vi "File list dialog.vi"(10 "Filters":string[](array[string])=["All files (*.*)|*.*"], 11 "File list in":path[](array[path])) -> (2 "Canceled?":bool, 3 "File list out":path[](array[path]))   [LabVIEW 2011, in "COSYLib.lvlib"]
doc: "Lets the user select a set of files.\nTo let the user select files of a specific type, use the <B>Filters</B> terminal. This is an array of strings of the format \"My Files (*.my)|*.my\"."
uses:
  COSYLib.lvlib
  <vilib>/Utility/miscctls.llb/LVPointTypeDef.ctl
panel:
  in  "Browse button":bool
  in  "Files of type:":string(combo)
  in  "Remove file":bool
  in  "Remove all":bool
  in  "Add all":bool
  in  "Add file":bool
  in  "Files":i32[](listbox)
  in  "Path":path
  in  "Selected files":i32[](listbox)
  out "Resized?":bool
  in  "Cancel":bool
  in  "OK":bool
  # "File Browser"
  # "Selected Files"
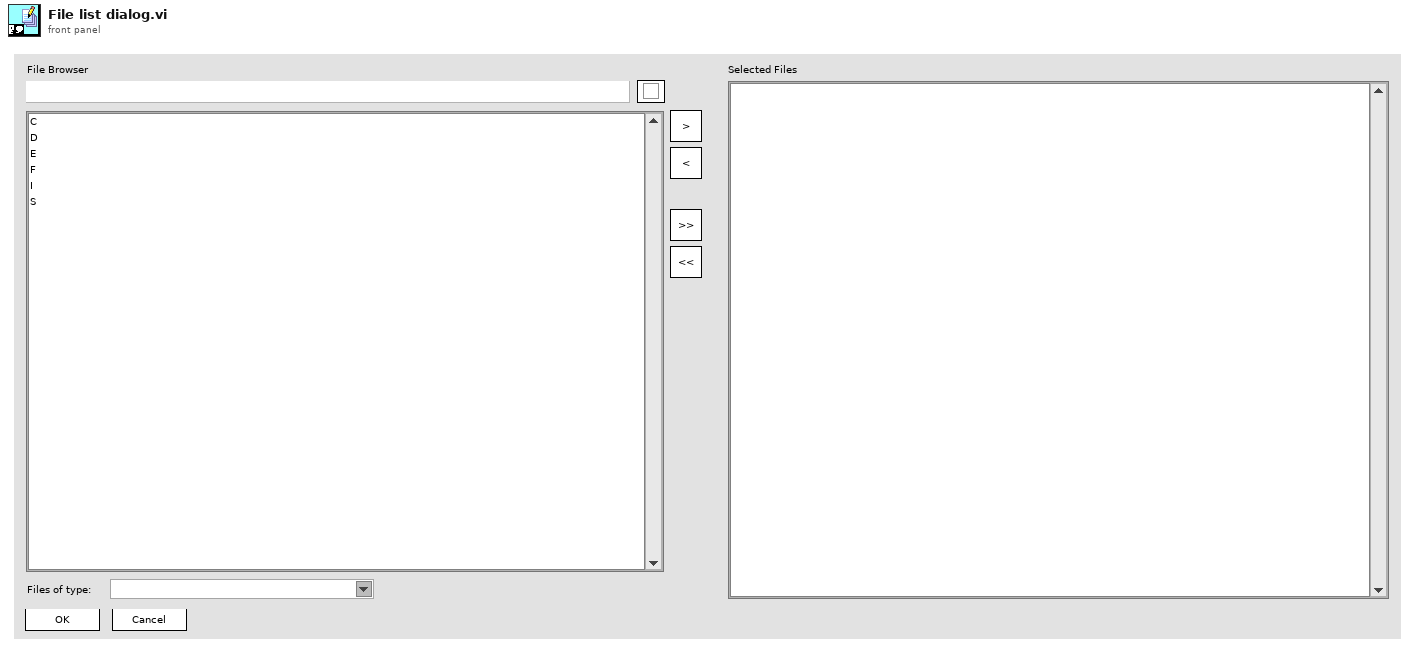
[diagram p1: front panel]
types:
  T1 = typedef "eventvkey.ctl" = enum16{"ASCII", "Enter", "Return", "Shift", "Ctrl", "Alt", "Cmd", "Opt", "Caps", "NumLock", "Clear", "Break", "Up", "Down", "Left", "Right", "Insert", "Delete", "Home", "End", "PageUp", "PageDown", "Escape", "Help", "Pause", "ScrollLock", "F1", "F2", "F3", "F4", "F5", "F6", "F7", "F8", "F9", "F10", "F11", "F12", "F13", "F14", "F15", "F16", "F17", "F18", "F19", "F20", "F21", "F22", "F23", "F24", "Play", "VolumeUp", "VolumeDown", "Mute", "Two Byte Char"}
  T2 = typedef "LVPointTypeDef.ctl" = cluster{"Horizontal":i16, "Vertical":i16}
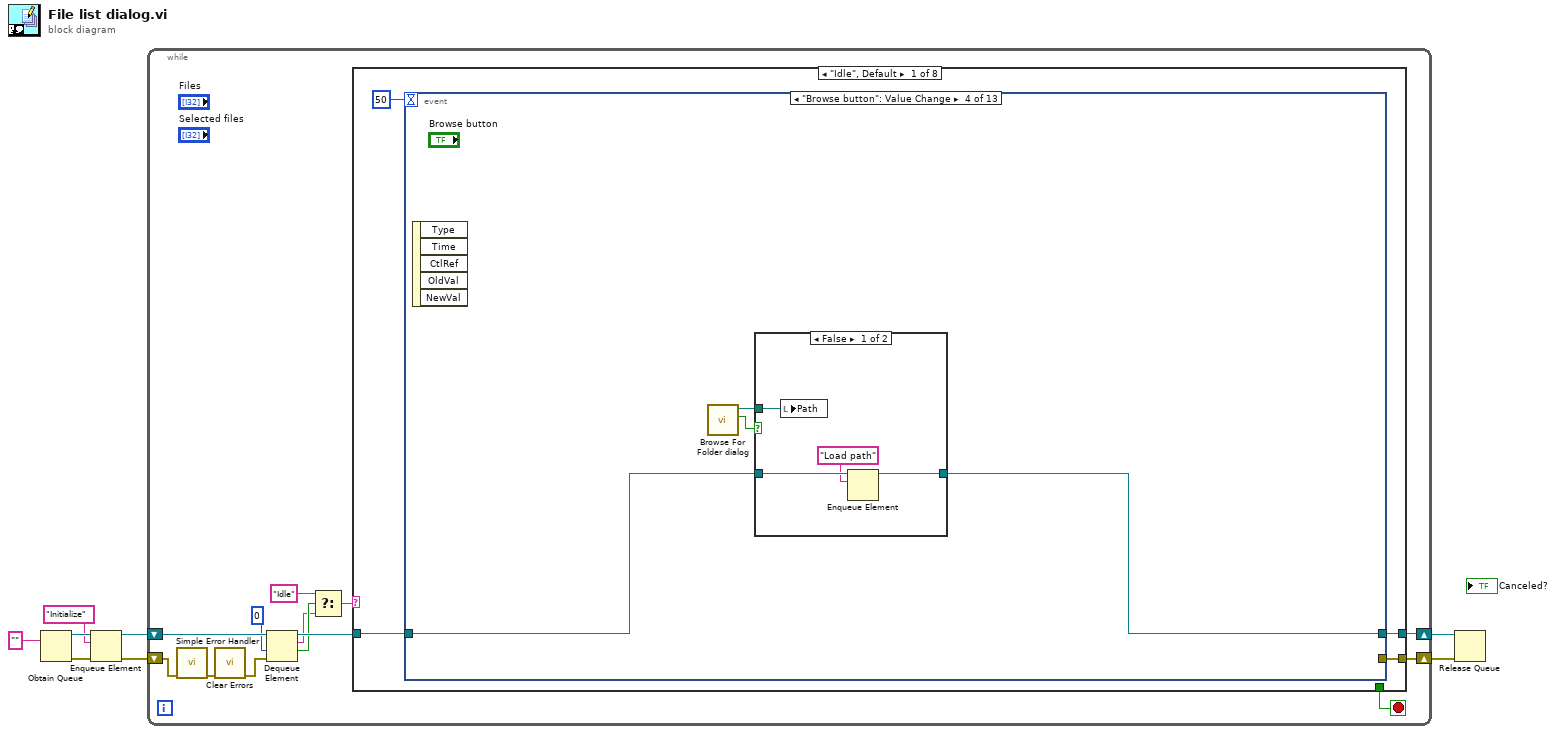
[diagram p0: block diagram]
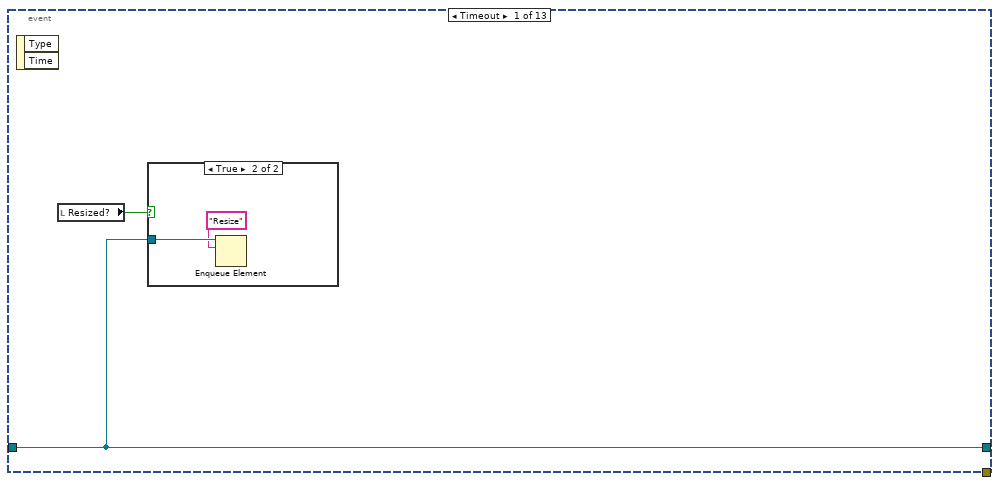
[diagram p2: hidden frame]
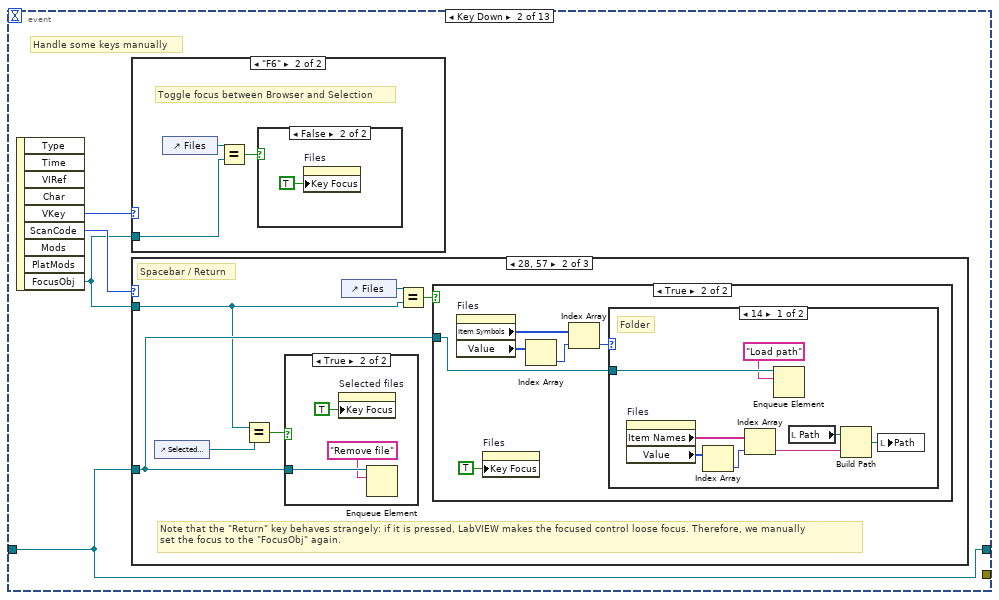
[diagram p4: hidden frame]
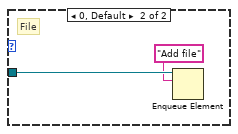
[diagram p8: hidden frame]
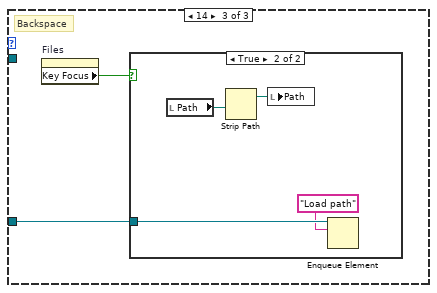
[diagram p9: hidden frame]
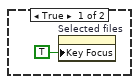
[diagram p12: hidden frame]
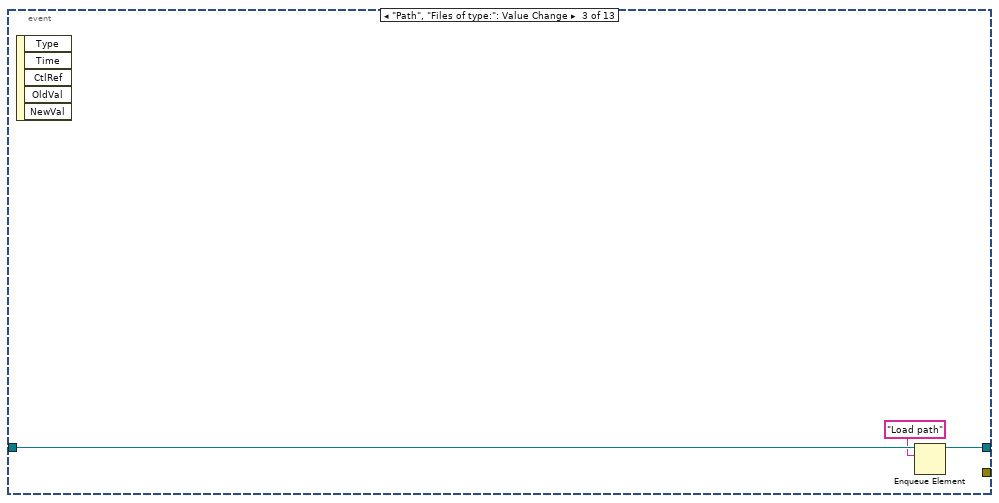
[diagram p13: hidden frame]
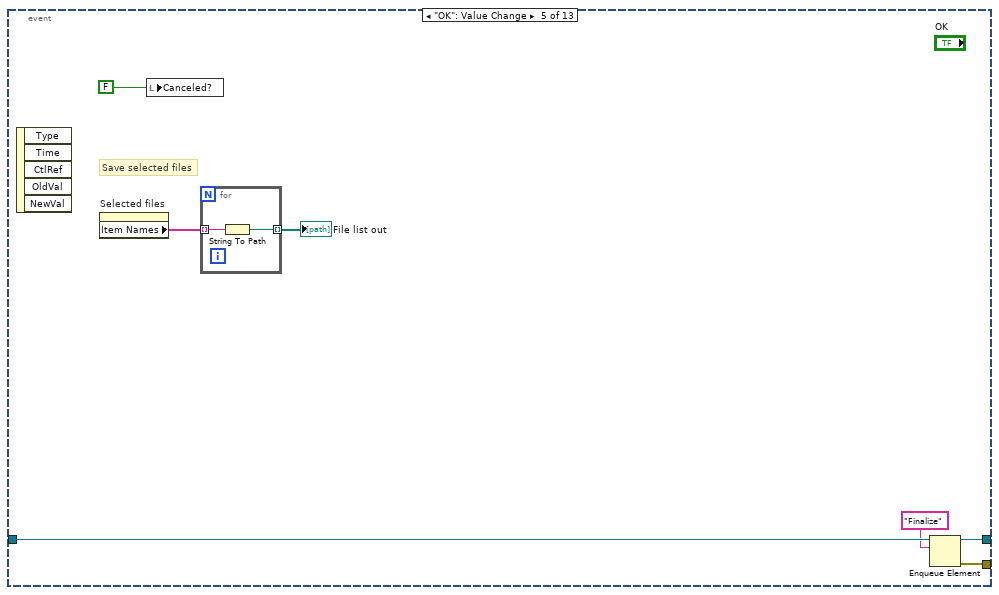
[diagram p15: hidden frame]
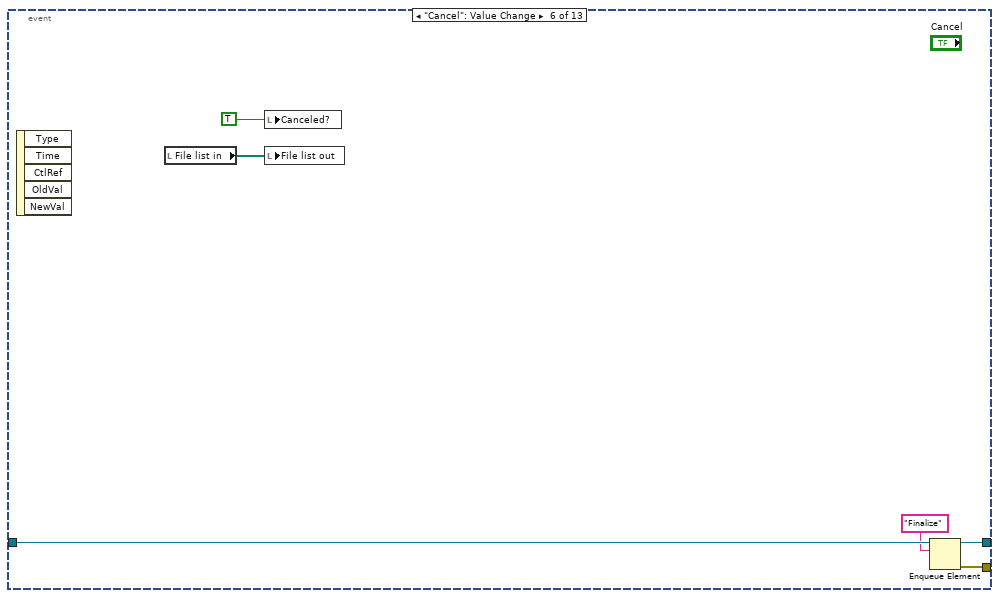
[diagram p16: hidden frame]
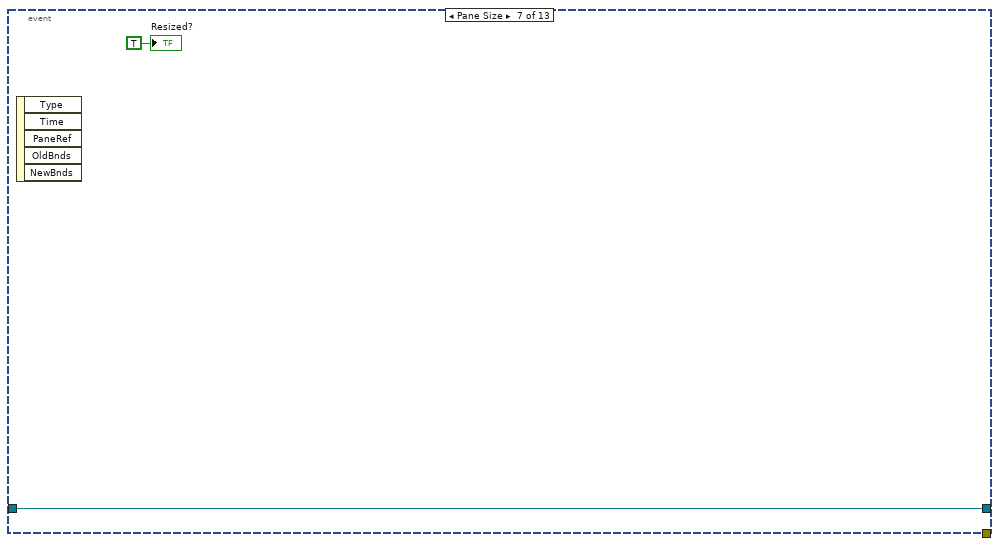
[diagram p17: hidden frame]
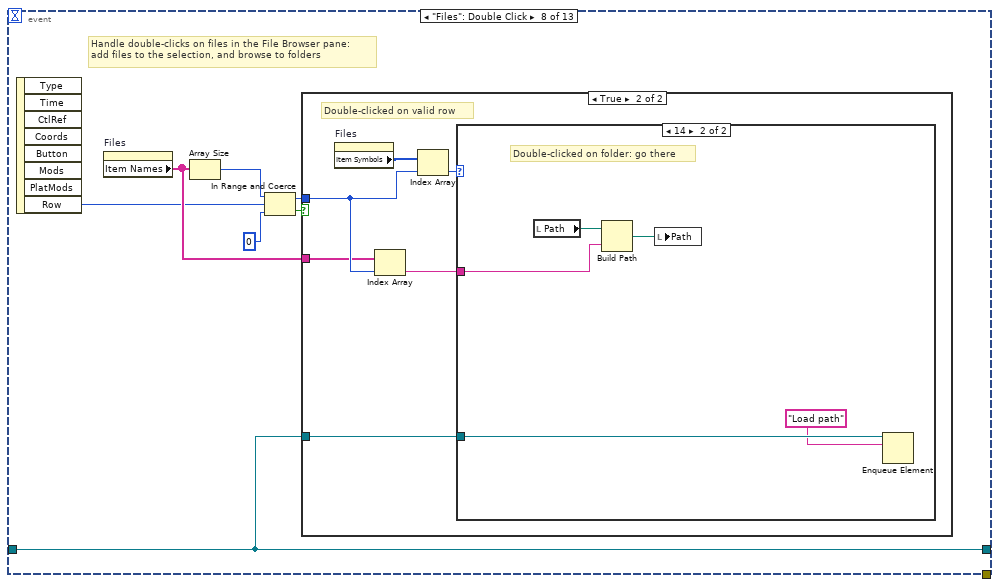
[diagram p18: hidden frame]
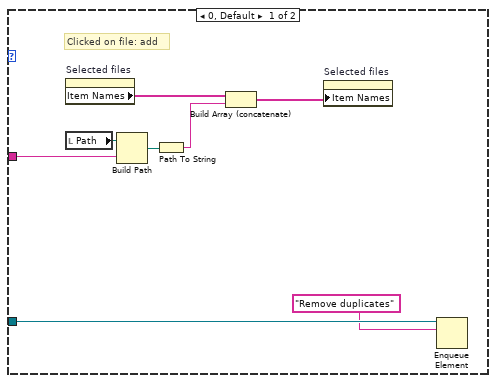
[diagram p20: hidden frame]
diagram:
  n1 = Obtain Queue(element data type="") -> (queue out=w7:refnum<queue>, error out=w6:errorcluster)  [unwired: 4 in, 1 out]
  n2 = Enqueue Element(queue=w7, element="Initialize", error in (no error)=w6) -> (queue out=w4:refnum<queue>, error out=w3:errorcluster)  [unwired: 1 in, 1 out]
  n3 = while {
    shift-right: [w10] -> w2
    shift-left: w3 -> [w20]
    shift-right: [w9] -> w1
    shift-left: w4 -> [w19]
    stop <- w21 stop-if-true
    n4 = call <vilib>:"Simple Error Handler.vi"("error in (no error)"=w20) -> ("error out"=w12:errorcluster)  [unwired: 4 in, 4 out]
    n5 = call <vilib>:"Clear Errors.vi"("error in (no error)"=w12) -> ("error out"=w11:errorcluster)  [unwired: 6 in]
    n6 = Dequeue Element(queue=w19, timeout in ms (-1)=0, error in (no error)=w11) -> (queue out=w17:refnum<queue>, element=w14:string, timed out?=w15:bool)  [unwired: 1 out]
    n7 = Select(t="Idle", s=w15, f=w14) -> (s? t:f=w18:string)
    n8 = case shown="\"Idle\", Default" w18 {
      tunnel: [_ _ TRUE _ _ _ _ _] -> w21
      tunnel: w17 -> [w25 w187 w199 w204 w231 w258 w284 w290]
      tunnel: [w24 _ _ _ _ _ _ _] -> w10
      tunnel: [w22 w177 w199 w204 w231 w249 w284 w290] -> w9
      frame "Idle", Default {
        n9 = event shown="[3] \"Browse button\": Value Change" {
          selector: _ -> [_ _ _ _ _ _ _ _ _ _ _ _ _]
          dyn-events: _ -> [_ _ _ _ _ _ _ _ _ _ _ _ _]
          timeout: 50 -> [_ _ _ _ _ _ _ _ _ _ _ _ _]
          tunnel: w25 -> [w26 w31 w72 w76 w88 w93 w98 w99 w131 w136 w146 w166 w169]
          tunnel: [_ _ _ _ w86 w95 _ _ _ _ _ _ _] -> w24
          tunnel: [w26 w31 w71 w75 w84 w94 w98 w99 w131 w136 w138 w165 w168] -> w22
          event Timeout {
            n10 = event-data() -> ()  [unwired: 1 in, 2 out]
            n11 = local read "Resized?"() -> (w27:bool)
            n12 = case shown="True" w27 {
              tunnel: w26 -> [_ w29]
              frame False {
              }
              frame True {
                n13 = Enqueue Element(queue=w29, element="Resize") -> ()  [unwired: 2 in, 3 out]
              }
            }
          }
          event Key Down {
            # "Handle some keys manually"
            n14 = event-data() -> ("VKey"=w33:T1, "ScanCode"=w32:i16, "FocusObj"=w30:refnum<vi>)  [unwired: 1 in, 6 out]
            n15 = case shown="\"F6\"" w33 {
              tunnel: w30 -> [_ w65]
              frame Default {
              }
              frame "F6" {
                # "Toggle focus between Browser and Selection"
                n16 = control-ref of="Files"() -> (w67:refnum<vi>)
                n17 = Equal?(x=w67, y=w65) -> (x = y?=w66:bool)
                n18 = case shown="False" w66 {
                  frame True {
                    n19 = property on="Selected files" class="LstBox (strict)"("Key Focus"=TRUE) -> ()  [unwired: 2 in, 2 out]
                  }
                  frame False {
                    n20 = property on="Files" class="LstBox (strict)"("Key Focus"=TRUE) -> ()  [unwired: 2 in, 2 out]
                  }
                }
              }
            }
            n21 = case shown="28, 57" w32 {
              tunnel: w31 -> [_ w39 w59]
              tunnel: w30 -> [_ w34 _]
              frame Default {
              }
              frame 28, 57 {
                # "Note that the \"Return\" key behaves strangely: if it is pressed, LabVIEW makes the focused control loose focus. Therefore, we manually\nset the focus to the \"FocusObj\" again."
                # "Spacebar / Return"
                n22 = control-ref of="Selected files"() -> (w35:refnum<vi>)
                n23 = Equal?(x=w34, y=w35) -> (x = y?=w36:bool)
                n24 = case shown="True" w36 {
                  tunnel: w39 -> [_ w42]
                  frame False {
                  }
                  frame True {
                    n25 = property on="Selected files" class="LstBox (strict)"("Key Focus"=TRUE) -> ()  [unwired: 2 in, 2 out]
                    n26 = Enqueue Element(queue=w42, element="Remove file") -> ()  [unwired: 2 in, 3 out]
                  }
                }
                n27 = control-ref of="Files"() -> (w37:refnum<vi>)
                n28 = Equal?(x=w37, y=w34) -> (x = y?=w38:bool)
                n29 = case shown="True" w38 {
                  tunnel: w39 -> [_ w46]
                  frame False {
                  }
                  frame True {
                    n30 = property on="Files" class="LstBox (strict)"() -> ("Item Symbols"=w48:i32[], "Value"=w45:i32[])  [unwired: 2 in, 2 out]
                    n31 = property on="Files" class="LstBox (strict)"("Key Focus"=TRUE) -> ()  [unwired: 2 in, 2 out]
                    n32 = Index Array(array=w45) -> (element=w44:i32)  [unwired: 1 in]
                    n33 = Index Array(array=w48, index=w44) -> (element=w47:i32)
                    n34 = case shown="14" w47 {
                      tunnel: w46 -> [w56 w58]
                      frame 14 {
                        # "Folder"
                        n35 = property on="Files" class="LstBox (strict)"() -> ("Item Names"=w52:string[], "Value"=w50:i32[])  [unwired: 2 in, 2 out]
                        n36 = Index Array(array=w50) -> (element=w49:i32)  [unwired: 1 in]
                        n37 = Index Array(array=w52, index=w49) -> (element=w51:string)
                        n38 = Enqueue Element(queue=w56, element="Load path") -> ()  [unwired: 2 in, 3 out]
                        n39 = local read "Path"() -> (w55:path)
                        n40 = Build Path(base path=w55, name or relative path=w51) -> (appended path=w54:path)
                        n41 = local write "Path"(w54) -> ()
                      }
                      frame 0, Default {
                        # "File"
                        n42 = Enqueue Element(queue=w58, element="Add file") -> ()  [unwired: 2 in, 3 out]
                      }
                    }
                  }
                }
              }
              frame 14 {
                # "Backspace"
                n43 = property on="Files" class="LstBox (strict)"() -> ("Key Focus"=w60:bool)  [unwired: 2 in, 2 out]
                n44 = case shown="True" w60 {
                  tunnel: w59 -> [_ w62]
                  frame False {
                  }
                  frame True {
                    n45 = local read "Path"() -> (w64:path)
                    n46 = Strip Path(path=w64) -> (stripped path=w63:path)  [unwired: 1 out]
                    n47 = local write "Path"(w63) -> ()
                    n48 = Enqueue Element(queue=w62, element="Load path") -> ()  [unwired: 2 in, 3 out]
                  }
                }
              }
            }
          }
          event "Path", "Files of type:": Value Change {
            n49 = event-data() -> ()  [unwired: 1 in, 5 out]
            n50 = Enqueue Element(queue=w72, element="Load path") -> (queue out=w71:refnum<queue>)  [unwired: 2 in, 2 out]
          }
          event "Browse button": Value Change {
            n51 = event-data() -> ()  [unwired: 1 in, 5 out]
            n52 = call "Browse For Folder dialog.vi"() -> ("Cancelled?"=w74:bool, "Selected path"=w73:path)  [unwired: 9 in, 1 out]
            n53 = case shown="False" w74 {
              tunnel: w76 -> [w80 w81]
              tunnel: [w79 w81] -> w75
              tunnel: w73 -> [w77 _]
              frame False {
                n54 = local write "Path"(w77) -> ()
                n55 = Enqueue Element(queue=w80, element="Load path") -> (queue out=w79:refnum<queue>)  [unwired: 2 in, 2 out]
              }
              frame True {
              }
            }
          }
          event "OK": Value Change {
            # "Save selected files"
            n56 = event-data() -> ()  [unwired: 1 in, 5 out]
            n57 = property on="Selected files" class="LstBox (strict)"() -> ("Item Names"=w83:string[])  [unwired: 2 in, 2 out]
            n58 = local write "Canceled?"(FALSE ("Canceled?")) -> ()
            n59 = for {
              tunnel: w83 -> [w90] mode=indexing
              tunnel: [w89] -> w82 mode=indexing
              n60 = String To Path(string=w90) -> (path=w89:path)
            }
            "File list out" <- w82
            n61 = Enqueue Element(queue=w88, element="Finalize") -> (queue out=w84:refnum<queue>, error out=w86:errorcluster)  [unwired: 2 in, 1 out]
          }
          event "Cancel": Value Change {
            n62 = event-data() -> ()  [unwired: 1 in, 5 out]
            n63 = local read "File list in"() -> (w91:path[])
            n64 = local write "Canceled?"(TRUE ("Canceled?")) -> ()
            n65 = local write "File list out"(w91) -> ()
            n66 = Enqueue Element(queue=w93, element="Finalize") -> (queue out=w94:refnum<queue>, error out=w95:errorcluster)  [unwired: 2 in, 1 out]
          }
          event Pane Size {
            n67 = event-data() -> ()  [unwired: 1 in, 5 out]
            "Resized?" <- TRUE ("Resized?")
          }
          event "Files": Double Click {
            # "Handle double-clicks on files in the File Browser pane:\nadd files to the selection, and browse to folders"
            n68 = event-data() -> ("Row"=w100:i32)  [unwired: 1 in, 7 out]
            n69 = property on="Files" class="LstBox (strict)"() -> ("Item Names"=w102:string[])  [unwired: 2 in, 2 out]
            n70 = Array Size(array=w102) -> (size(s)=w101:i32)
            n71 = In Range and Coerce(upper limit=w101, x=w100, lower limit=0 ("upper limit")) -> (coerced(x)=w104:i32, In Range?=w105:bool)
            n72 = case shown="True" w105 {
              tunnel: w104 -> [_ w109]
              tunnel: w102 -> [_ w108]
              tunnel: w99 -> [_ w106]
              frame False {
                # "Double-clicked on an invalid/empty row"
              }
              frame True {
                # "Double-clicked on valid row"
                n73 = property on="Files" class="LstBox (strict)"() -> ("Item Symbols"=w111:i32[])  [unwired: 2 in, 2 out]
                n74 = Index Array(array=w108, index=w109) -> (element=w107:string)
                n75 = Index Array(array=w111, index=w109) -> (element=w110:i32)
                n76 = case shown="14" w110 {
                  tunnel: w107 -> [w116 w123]
                  tunnel: w106 -> [w113 w121]
                  frame 0, Default {
                    # "Clicked on file: add"
                    n77 = property on="Selected files" class="LstBox (strict)"() -> ("Item Names"=w119:string[])  [unwired: 2 in, 2 out]
                    n78 = local read "Path"() -> (w117:path)
                    n79 = Build Path(base path=w117, name or relative path=w116) -> (appended path=w115:path)
                    n80 = Path To String(path=w115) -> (string=w114:string)
                    n81 = Build Array (concatenate)(w119, w114) -> (w118:string[])
                    n82 = property on="Selected files" class="LstBox (strict)"("Item Names"=w118) -> ()  [unwired: 2 in, 2 out]
                    n83 = Enqueue Element(queue=w113, element="Remove duplicates") -> ()  [unwired: 2 in, 3 out]
                  }
                  frame 14 {
                    # "Double-clicked on folder: go there"
                    n84 = local read "Path"() -> (w124:path)
                    n85 = Build Path(base path=w124, name or relative path=w123) -> (appended path=w122:path)
                    n86 = local write "Path"(w122) -> ()
                    n87 = Enqueue Element(queue=w121, element="Load path") -> ()  [unwired: 2 in, 3 out]
                  }
                }
              }
            }
          }
          event "Selected files": Double Click {
            # "Remove the file that was double-clicked from the \"Selected files\""
            n88 = event-data() -> ("Row"=w125:i32)  [unwired: 1 in, 7 out]
            n89 = property on="Selected files" class="LstBox (strict)"() -> ("Item Names"=w129:string[])  [unwired: 2 in, 2 out]
            n90 = Array Size(array=w129) -> (size(s)=w128:i32)
            n91 = In Range and Coerce(upper limit=w128, x=w125, lower limit=0 ("upper limit")) -> (coerced(x)=w126:i32, In Range?=w127:bool)
            n92 = case shown="True" w127 {
              tunnel: w126 -> [_ w134]
              frame False {
                # "Double-clicked on an invalid/empty row"
              }
              frame True {
                # "Double-clicked on valid row"
                n93 = property on="Selected files" class="LstBox (strict)"() -> ("Item Names"=w133:string[])  [unwired: 2 in, 2 out]
                n94 = Delete From Array(array=w133, index=w134) -> (array with subset deleted=w132:string[])  [unwired: 1 in, 1 out]
                n95 = property on="Selected files" class="LstBox (strict)"("Item Names"=w132) -> ()  [unwired: 2 in, 2 out]
              }
            }
          }
          event "Remove all": Value Change {
            n96 = event-data() -> ()  [unwired: 1 in, 5 out]
            n97 = property on="Selected files" class="LstBox (strict)"("Item Names"=string[] []) -> ()  [unwired: 2 in, 2 out]
          }
          event "Add all": Value Change {
            # "Add all files in the Browser to the \"Selected files\""
            n98 = event-data() -> ()  [unwired: 1 in, 5 out]
            n99 = property on="Files" class="LstBox (strict)"() -> ("Item Names"=w145:string[], "Item Symbols"=w144:i32[])  [unwired: 2 in, 2 out]
            n100 = local read "Path"() -> (w143:path)
            n101 = for {
              tunnel: w145 -> [w149] mode=indexing
              tunnel: w144 -> [w151] mode=indexing
              tunnel: w143 -> [w150]
              shift-right: [w147] -> w139
              shift-left: string[] [] -> [w148]
              n102 = case shown="0, Default" w151 {
                tunnel: w150 -> [w157 _]
                tunnel: w149 -> [w156 _]
                tunnel: w148 -> [w155 w163]
                tunnel: [w154 w163] -> w147
                frame 0, Default {
                  # "Add files only"
                  n103 = Build Path(base path=w157, name or relative path=w156) -> (appended path=w153:path)
                  n104 = Not A Number/Path/Refnum?(number/path/refnum=w153) -> (NaN/Path/Refnum?=w152:bool)
                  n105 = case shown="False" w152 {
                    tunnel: w153 -> [w161 _]
                    tunnel: w155 -> [w159 w162]
                    tunnel: [w158 w162] -> w154
                    frame False {
                      n106 = Path To String(path=w161) -> (string=w160:string)
                      n107 = Build Array (concatenate)(w159, w160) -> (w158:string[])
                    }
                    frame True {
                      # "Skip invalid paths"
                    }
                  }
                }
                frame 14 {
                  # "Ignore folders"
                }
              }
            }
            n108 = property on="Selected files" class="LstBox (strict)"() -> ("Item Names"=w141:string[])  [unwired: 2 in, 2 out]
            n109 = Build Array (concatenate)(w141, w139) -> (w140:string[])
            n110 = property on="Selected files" class="LstBox (strict)"("Item Names"=w140) -> ()  [unwired: 2 in, 2 out]
            n111 = Enqueue Element(queue=w146, element="Remove duplicates") -> (queue out=w138:refnum<queue>)  [unwired: 2 in, 2 out]
          }
          event "Add file": Value Change {
            n112 = event-data() -> ()  [unwired: 1 in, 5 out]
            n113 = Enqueue Element(queue=w166, element="Add file") -> (queue out=w165:refnum<queue>)  [unwired: 2 in, 2 out]
          }
          event "Remove file": Value Change {
            n114 = event-data() -> ()  [unwired: 1 in, 5 out]
            n115 = Enqueue Element(queue=w169, element="Remove file") -> (queue out=w168:refnum<queue>)  [unwired: 2 in, 2 out]
          }
        }
      }
      frame "Initialize" {
        w186 = T2 {"Horizontal"=0, "Vertical"=0} ("Origin")
        # "Select first filter by default"
        # "Load filters"
        # "Load input list; by default, we start with the path of the last file in the list"
        n116 = property on="File Browser Pane" class="Pane"("Origin"=w186) -> ()  [unwired: 2 in, 2 out]
        n117 = property on="Selection Pane" class="Pane"("Origin"=w186) -> ()  [unwired: 2 in, 2 out]
        n118 = for {
          tunnel: "Filters" -> [w194] mode=indexing
          tunnel: [w188] -> w173 mode=indexing
          n119 = Search/Split String(string=w194, search string/char (-)="|") -> (substring before match=w189:string, match + rest of string=w192:string)  [unwired: 1 in, 1 out]
          n120 = String Subset(string=w192, offset (0)=1) -> (substring=w190:string)  [unwired: 1 in]
          n121 = Bundle("Filter"=w189, "Filter"=w190) -> (w188:cluster{"Filter":string, "Filter":string})  [unwired: 1 in]
        }
        n122 = Reverse 1D Array(array="File list in") -> (reversed array=w182:path[])
        n123 = for {
          tunnel: "File list in" -> [w198] mode=indexing
          tunnel: [w197] -> w183 mode=indexing
          n124 = Path To String(path=w198) -> (string=w197:string)
        }
        n125 = Index Array(array=w182) -> (element=w181:path)  [unwired: 1 in]
        n126 = Strip Path(path=w181) -> (stripped path=w179:path)  [unwired: 1 out]
        n127 = property on="Files" class="LstBox (strict)"("Key Focus"=TRUE) -> ()  [unwired: 2 in, 2 out]
        n128 = Not A Number/Path/Refnum?(number/path/refnum=w179) -> (NaN/Path/Refnum?=w180:bool)
        n129 = case shown="True" w180 {
          tunnel: w179 -> [w195 _]
          tunnel: [w195 path ""] -> w178
          frame False {
          }
          frame True {
          }
        }
        n130 = property on="Selected files" class="LstBox (strict)"("Item Names"=w183) -> ()  [unwired: 2 in, 2 out]
        n131 = Index Array(array=w173) -> (element=w172:cluster{"Filter":string, "Filter":string})  [unwired: 1 in]
        n132 = local write "Path"(w178) -> ()
        n133 = Unbundle(w172) -> ("Filter"=w171:string)  [unwired: 1 out]
        n134 = property on="Files of type:" class="CmbBox"("Strings And Values[]"=w173, "Value"=w171) -> ()  [unwired: 2 in, 2 out]
        n135 = Enqueue Element(queue=w187, element="Resize") -> (queue out=w185:refnum<queue>)  [unwired: 2 in, 2 out]
        n136 = Enqueue Element(queue=w185, element="Load path") -> (queue out=w177:refnum<queue>)  [unwired: 2 in, 2 out]
      }
      frame "Finalize" {
      }
      frame "Resize" {
        # "When the panes are resized, we have to make some manual adjustments..."
        n137 = property on="File Browser Pane" class="Pane"() -> ("Width"=w214:u32, "Height"=w201:u32)  [unwired: 2 in, 2 out]
        n138 = Subtract(x=w214, y=u32 91) -> (x-y=w221:u32)
        n139 = Subtract(x=w214, y=u32 57) -> (x-y=w213:u32)
        n140 = Subtract(x=w201, y=u32 92) -> (x-y=w215:u32)
        n141 = property on="Path" class="Path"("Width"=w221) -> ()  [unwired: 2 in, 2 out]
        n142 = property on="Files" class="LstBox (strict)"("Width"=w213, "Height"=w215) -> ()  [unwired: 2 in, 2 out]
        n143 = Add(x=w213, y=u32 18) -> (x+y=w211:u32)
        n144 = Subtract(x=w201, y=u32 28) -> (x-y=w202:u32)
        n145 = property on="Files of type:" class="CmbBox"("Top"=w202) -> ()  [unwired: 2 in, 2 out]
        n146 = property on="Add file" class="Bool"("Left"=w211) -> ()  [unwired: 2 in, 2 out]
        n147 = property on="Remove file" class="Bool"("Left"=w211, "Top"=93 ("Position:Top")) -> ()  [unwired: 2 in, 2 out]
        n148 = property on="Add all" class="Bool"("Left"=w211, "Top"=155 ("Position:Top")) -> ()  [unwired: 2 in, 2 out]
        n149 = property on="Remove all" class="Bool"("Left"=w211, "Top"=192 ("Position:Top")) -> ()  [unwired: 2 in, 2 out]
        n150 = property on="Selection Pane" class="Pane"() -> ("Width"=w208:u32, "Height"=w207:u32)  [unwired: 2 in, 2 out]
        n151 = Subtract(x=w208, y=u32 25) -> (x-y=w206:u32)
        n152 = Subtract(x=w207, y=u32 35) -> (x-y=w205:u32)
        n153 = property on="Selected files" class="LstBox (strict)"("Width"=w206, "Height"=w205) -> ()  [unwired: 2 in, 2 out]
      }
      frame "Load path" {
        # "Add \"..\", but not\nto root path"
        # "> folders >"
        # "> files >"
        # "Fill the \"Files\" listbox with all files in the given path"
        n154 = Not Equal?(x="Path", y=path "") -> (x != y?=w225:bool)
        n155 = List Folder(path="Path") -> (folder names=w228:string[])  [unwired: 3 in, 3 out]
        n156 = List Folder(path="Path", pattern="Files of type:") -> (filenames=w229:string[], error out=w230:errorcluster)  [unwired: 2 in, 2 out]
        n157 = case shown="True" w225 {
          tunnel: w228 -> [w232 w236]
          tunnel: [w232 w235] -> w227
          frame False {
          }
          frame True {
            n158 = Insert Into Array(array=w236, index=0, new element=".." ("new element/subarray")) -> (w235:string[])
          }
        }
        n159 = case shown="No Error" w230 {
          tunnel: w229 -> [w239 _]
          tunnel: w227 -> [w246 _]
          frame No Error {
            # "Here we give all the folders a \"folder\" icon in the listbox"
            n160 = Array Size(array=w246) -> (size(s)=w245:i32)
            n161 = Array Size(array=w239) -> (size(s)=w241:i32)
            n162 = Build Array (concatenate)(w246, w239) -> (w247:string[])
            n163 = Initialize Array(14 ("element"), w245) -> (w244:i32[])
            n164 = Initialize Array(0 ("element"), w241) -> (w238:i32[])
            n165 = Build Array (concatenate)(w244, w238) -> (w242:i32[])
            n166 = property on="Files" class="LstBox (strict)"("Item Names"=w247, "Item Symbols"=w242, "Value"=i32[] [] ("Files")) -> ()  [unwired: 2 in, 2 out]
          }
          frame Error {
          }
        }
        n167 = call <vilib>:"Clear Errors.vi"("error in (no error)"=w230) -> ()  [unwired: 6 in, 1 out]
      }
      frame "Add file" {
        # "Add the files that have been selected in the Browser to the \"Selected files\""
        n168 = property on="Files" class="LstBox (strict)"() -> ("Item Names"=w250:string[], "Item Symbols"=w251:i32[])  [unwired: 2 in, 2 out]
        n169 = local read "Files"() -> (w257:i32[])
        n170 = local read "Path"() -> (w252:path)
        n171 = for {
          tunnel: w250 -> [w263]
          tunnel: w251 -> [w262]
          tunnel: w252 -> [w266]
          shift-right: [w264] -> w256
          shift-left: string[] [] -> [w265]
          tunnel: w257 -> [w261] mode=indexing
          n172 = Index Array(array=w263, index=w261) -> (element=w259:string)
          n173 = Index Array(array=w262, index=w261) -> (element=w260:i32)
          n174 = case shown="0, Default" w260 {
            tunnel: w266 -> [w272 _]
            tunnel: w265 -> [w271 w278]
            tunnel: [w270 w278] -> w264
            tunnel: w259 -> [w269 _]
            frame 0, Default {
              # "Add files only"
              n175 = Build Path(base path=w272, name or relative path=w269) -> (appended path=w267:path)
              n176 = Not A Number/Path/Refnum?(number/path/refnum=w267) -> (NaN/Path/Refnum?=w268:bool)
              n177 = case shown="True" w268 {
                tunnel: w267 -> [w276 _]
                tunnel: w271 -> [w274 w277]
                tunnel: [w273 w277] -> w270
                frame False {
                  n178 = Path To String(path=w276) -> (string=w275:string)
                  n179 = Build Array (concatenate)(w274, w275) -> (w273:string[])
                }
                frame True {
                  # "Skip invalid paths"
                }
              }
            }
            frame 14 {
              # "Ignore folders"
            }
          }
        }
        n180 = property on="Selected files" class="LstBox (strict)"() -> ("Item Names"=w254:string[])  [unwired: 2 in, 2 out]
        n181 = Build Array (concatenate)(w254, w256) -> (w255:string[])
        n182 = property on="Selected files" class="LstBox (strict)"("Item Names"=w255) -> ()  [unwired: 2 in, 2 out]
        n183 = Enqueue Element(queue=w258, element="Remove duplicates") -> (queue out=w249:refnum<queue>)  [unwired: 2 in, 2 out]
      }
      frame "Remove file" {
        # "Remove the files that are selected in the \"Selected files\" listbox"
        n184 = local read "Selected files"() -> (w280:i32[])
        n185 = property on="Selected files" class="LstBox (strict)"() -> ("Item Names"=w282:string[])  [unwired: 2 in, 2 out]
        n186 = Reverse 1D Array(array=w280) -> (reversed array=w281:i32[])
        n187 = for {
          tunnel: w281 -> [w286] mode=indexing
          shift-right: [w285] -> w283
          shift-left: w282 -> [w287]
          n188 = Delete From Array(array=w287, index=w286) -> (array with subset deleted=w285:string[])  [unwired: 1 in, 1 out]
        }
        n189 = property on="Selected files" class="LstBox (strict)"("Item Names"=w283, "Value"=i32[] [] ("Selected files")) -> ()  [unwired: 2 in, 2 out]
      }
      frame "Remove duplicates" {
        n190 = property on="Selected files" class="LstBox (strict)"() -> ("Item Names"=w289:string[])  [unwired: 2 in, 2 out]
        n191 = call "Remove duplicates from 1D String Array.vi"("Array"=w289) -> ("Array w/o duplicates"=w288:string[])
        n192 = property on="Selected files" class="LstBox (strict)"("Item Names"=w288) -> ()  [unwired: 2 in, 2 out]
      }
    }
  }
  n193 = Release Queue(queue=w1, error in (no error)=w2) -> ()  [unwired: 1 in, 3 out]
